vi "Initalize SR830(SubVI).vi"(0 "簇":T1={"initialize"=enum."SR830", "6221"={"6221 Resource"="GPIB0::24::INSTR", "Delta status"=FALSE, "电流"=0.0}, "SR830+6221"={"source"=0, "阻抗"=0.0, "量程入 4"=0, "量程入 3"=0, "量程入 2"=0, "量程入 1"=0, "SR830 2"=FALSE, "SR830 3"=FALSE, "SR830 4"=FALSE, "SR830 1"=FALSE, "VISA 1"="", "VISA 2"="", "VISA 3"="", "VISA 4"="", "量程"=enum."量程每次测量会判定"}, "2400"={"2400"=FALSE, "VISA"=""}, "ch"={"ch"=[], "current"=[], "change?"=[], "holding current\nwhen change ch?"=FALSE}, "Instrument"={"335 Resource"="GPIB0::24::INSTR", "Input (0:A)"=0, "Instrument Type"=enum."SVSM", "quantum design"=refnum, "Heater Output (1:1)"=1, "semaphore"=refnum, "TCP master instance"=refnum, "335 Status"=refnum, "M24C Resource"="GPIB0::24::INSTR", "4G supply"="GPIB0::24::INSTR", "Temp Status 24C"=refnum, "4g supply status"=refnum}, "Aborting"=refnum, "数据文件"=refnum} {"Instrument"."Input (0:A)" items=["A", "B"]; "Instrument"."Heater Output (1:1)" items=["1"=1, "2"=2]; "SR830+6221"."source" items=["SR830 1", "SR830 2", "SR830 3", "SR830 4"]}, 9 "字符串":string) -> (4 "输出簇":T1={"initialize"=enum."SR830", "6221"={"6221 Resource"="GPIB0::24::INSTR", "Delta status"=FALSE, "电流"=0.0}, "SR830+6221"={"source"=0, "阻抗"=0.0, "量程入 4"=0, "量程入 3"=0, "量程入 2"=0, "量程入 1"=0, "SR830 2"=FALSE, "SR830 3"=FALSE, "SR830 4"=FALSE, "SR830 1"=FALSE, "VISA 1"="", "VISA 2"="", "VISA 3"="", "VISA 4"="", "量程"=enum."量程每次测量会判定"}, "2400"={"2400"=FALSE, "VISA"=""}, "ch"={"ch"=[], "current"=[], "change?"=[], "holding current\nwhen change ch?"=FALSE}, "Instrument"={"335 Resource"="GPIB0::24::INSTR", "Input (0:A)"=0, "Instrument Type"=enum."SVSM", "quantum design"=refnum, "Heater Output (1:1)"=1, "semaphore"=refnum, "TCP master instance"=refnum, "335 Status"=refnum, "M24C Resource"="GPIB0::24::INSTR", "4G supply"="GPIB0::24::INSTR", "Temp Status 24C"=refnum, "4g supply status"=refnum}, "Aborting"=refnum, "数据文件"=refnum} {"Instrument"."Input (0:A)" items=["A", "B"]; "Instrument"."Heater Output (1:1)" items=["1"=1, "2"=2]; "SR830+6221"."source" items=["SR830 1", "SR830 2", "SR830 3", "SR830 4"]})   [LabVIEW 2019, in "SubVI.lvlib"]
uses:
  SubVI.lvlib
  lib/Keithley 622x/Configure/6221 Wave/Typedefs/KE6221 -- Wave Sine Wave Params.ctl
  lib/Keithley 622x/Configure/6221 Wave/Low Level/Typedefs/KE6221 -- Wave Frequency.ctl
  lib/Keithley 622x/Configure/6221 Wave/Low Level/Typedefs/KE6221 -- Wave Amplitude.ctl
  lib/Keithley 622x/Configure/Source/Typedefs/KE622x -- Current Level.ctl
  lib/Keithley 622x/Configure/6221 Wave/Low Level/Typedefs/KE6221 -- Wave Ranging Mode.ctl
  lib/Keithley 622x/Configure/Source/Typedefs/KE622x -- Current Ranges.ctl
  lib/Keithley 622x/Configure/6221 Wave/Low Level/Typedefs/KE6221 -- Wave Playback Mode.ctl
  lib/Keithley 622x/Configure/6221 Wave/Low Level/Typedefs/KE6221 -- Wave Playback Time.ctl
  lib/Keithley 622x/Configure/6221 Wave/Low Level/Typedefs/KE6221 -- Wave Playback Num Cycles.ctl
  lib/Keithley 622x/Configure/6221 Wave/Low Level/Typedefs/KE6221 -- Wave Phase Marker.ctl
  lib/Keithley 622x/Configure/Trigger/Low Level/Typedefs/KE622x -- Trig Link Line.ctl
  config.ctl
  <vilib>/NI/Modbus Library/API/Master/Modbus Master.lvclass
  initialize.ctl
  Instrument.ctl
  Instrument Type.ctl
  lib/QDInstrument.dll
  335 state.ctl
  lib/Keithley 622x/Configure/6221 Wave/Low Level/Typedefs/KE6221 -- Wave Type.ctl
  lib/Keithley 622x/Keithley 622x.lvlib
panel:
  in  "同步 3":bool
  in  "同步 2":bool
  in  "同步":bool
  in  "6221(SR830做源可忽略）":T17={"Sine Wave Params In"={"Frequency (Hz)"=1000.0, "Amplitude (A)"=0.001, "Offset (A)"=0.0, "Ranging Mode"=enum."Best", "Fixed Range"=enum."2mA", "Playback Mode"=enum."Time", "Time (s)"=999999.999, "Num Cycles"=1.0, "Phase\nMarker?"=FALSE, "Phase Marker (deg)"=180.0, "Trig Link Line"=enum."1"}, "RMS Amplitude (A)"=0.001, "6221 resource"=""} {"RMS Amplitude (A)" min=2e-12 max=0.105 format="%.3p"; "Sine Wave Params In"."Offset (A)" min=-0.105 max=0.105 format="%.4p"; "Sine Wave Params In"."Num Cycles" min=0.001 max=99999999900.0 format="%.3p"; "Sine Wave Params In"."Time (s)" min=1e-07 max=999999.999 format="%.3p"; "Sine Wave Params In"."Phase Marker (deg)" min=0.0 max=360.0 format="%.3f"; "Sine Wave Params In"."Amplitude (A)" min=2e-12 max=0.105 format="%.3p"; "Sine Wave Params In"."Frequency (Hz)" min=0.001 max=100000.0 format="%.3p"}
  in  "仪器设置":T18={"ID Query"=FALSE, "Reset"=FALSE, "VISA 1"="", "VISA 2"="", "VISA 3"="", "VISA 4"="", "Sensitivity 2"=-1, "Sensitivity 1"=-1, "量程"=enum."量程每次测量会判定", "SR830源配合的阻抗（6221做源可忽略）"=0.0, "SR830 2"=FALSE, "SR830 3"=FALSE, "SR830 4"=FALSE, "Sensitivity 3"=-1, "Sensitivity 4"=-1, "source"=0, "SR830 1"=FALSE} {"source" items=["SR830 1", "SR830 2", "SR830 3", "SR830 4", "6221"]; "Sensitivity 4" items=["Auto Gain"=-1, "2 nV/fA"=0, "5 nV/fA"=1, "10 nV/fA"=2, "20 nV/fA"=3, "50 nV/fA"=4, "100 nV/fA"=5, "200 nV/fA"=6, "500 nV/fA"=7, "1 uV/pA"=8, "2 uV/pA"=9, "5 uV/pA"=10, "10 uV/pA"=11, "20 uV/pA"=12, "50 uV/pA"=13, "100 uV/pA"=14, "200 uV/pA"=15, "500 uV/pA"=16, "1 mV/nA"=17, "2 mV/nA"=18, "5 mV/nA"=19, "10 mV/nA"=20, "20 mV/nA"=21, "50 mV/nA"=22, "100 mV/nA"=23, "200 mV/nA"=24, "500 mV/mA"=25, "1 V/uA"=26]; "Sensitivity 3" items=["Auto Gain"=-1, "2 nV/fA"=0, "5 nV/fA"=1, "10 nV/fA"=2, "20 nV/fA"=3, "50 nV/fA"=4, "100 nV/fA"=5, "200 nV/fA"=6, "500 nV/fA"=7, "1 uV/pA"=8, "2 uV/pA"=9, "5 uV/pA"=10, "10 uV/pA"=11, "20 uV/pA"=12, "50 uV/pA"=13, "100 uV/pA"=14, "200 uV/pA"=15, "500 uV/pA"=16, "1 mV/nA"=17, "2 mV/nA"=18, "5 mV/nA"=19, "10 mV/nA"=20, "20 mV/nA"=21, "50 mV/nA"=22, "100 mV/nA"=23, "200 mV/nA"=24, "500 mV/mA"=25, "1 V/uA"=26]; "Sensitivity 1" items=["Auto Gain"=-1, "2 nV/fA"=0, "5 nV/fA"=1, "10 nV/fA"=2, "20 nV/fA"=3, "50 nV/fA"=4, "100 nV/fA"=5, "200 nV/fA"=6, "500 nV/fA"=7, "1 uV/pA"=8, "2 uV/pA"=9, "5 uV/pA"=10, "10 uV/pA"=11, "20 uV/pA"=12, "50 uV/pA"=13, "100 uV/pA"=14, "200 uV/pA"=15, "500 uV/pA"=16, "1 mV/nA"=17, "2 mV/nA"=18, "5 mV/nA"=19, "10 mV/nA"=20, "20 mV/nA"=21, "50 mV/nA"=22, "100 mV/nA"=23, "200 mV/nA"=24, "500 mV/mA"=25, "1 V/uA"=26]; "Sensitivity 2" items=["Auto Gain"=-1, "2 nV/fA"=0, "5 nV/fA"=1, "10 nV/fA"=2, "20 nV/fA"=3, "50 nV/fA"=4, "100 nV/fA"=5, "200 nV/fA"=6, "500 nV/fA"=7, "1 uV/pA"=8, "2 uV/pA"=9, "5 uV/pA"=10, "10 uV/pA"=11, "20 uV/pA"=12, "50 uV/pA"=13, "100 uV/pA"=14, "200 uV/pA"=15, "500 uV/pA"=16, "1 mV/nA"=17, "2 mV/nA"=18, "5 mV/nA"=19, "10 mV/nA"=20, "20 mV/nA"=21, "50 mV/nA"=22, "100 mV/nA"=23, "200 mV/nA"=24, "500 mV/mA"=25, "1 V/uA"=26]}
  out "错误输出":errorcluster
  in  "滤波设置 4":T19={"Time Constant "=8, "Low Pass Filter Slope "=1, "Enable Sync Filter "=TRUE} {"Low Pass Filter Slope" items=["6 dB/oct", "12 dB/oct", "18 db/oct", "24 dB/oct"]; "Time Constant" items=["10 us", "30 us", "100 us", "300 us", "1 ms", "3 ms", "10 ms", "30 ms", "100 ms", "300 ms", "1 s", "3 s", "10 s", "30 s", "100 s", "300 s", "1 ks", "3 ks", "10 ks", "30 ks"]}
  in  "滤波设置 3":T19={"Time Constant "=8, "Low Pass Filter Slope "=1, "Enable Sync Filter "=TRUE} {"Low Pass Filter Slope" items=["6 dB/oct", "12 dB/oct", "18 db/oct", "24 dB/oct"]; "Time Constant" items=["10 us", "30 us", "100 us", "300 us", "1 ms", "3 ms", "10 ms", "30 ms", "100 ms", "300 ms", "1 s", "3 s", "10 s", "30 s", "100 s", "300 s", "1 ks", "3 ks", "10 ks", "30 ks"]}
  in  "滤波设置 2":T19={"Time Constant "=8, "Low Pass Filter Slope "=1, "Enable Sync Filter "=TRUE} {"Low Pass Filter Slope" items=["6 dB/oct", "12 dB/oct", "18 db/oct", "24 dB/oct"]; "Time Constant" items=["10 us", "30 us", "100 us", "300 us", "1 ms", "3 ms", "10 ms", "30 ms", "100 ms", "300 ms", "1 s", "3 s", "10 s", "30 s", "100 s", "300 s", "1 ks", "3 ks", "10 ks", "30 ks"]}
  in  "参考信号 4":T20={"Reference Source"=1, "External Reference Trigger  "=0, "Detection Harmonic Number "=1.0, "Manual Phase (Degree)"=0.0, "Auto Phase "=FALSE, "Sine Output Amplitude (V)"=1.0, "Internal Reference Frequency (Hz)"=13.0} {"External Reference Trigger" items=["Sine Zero Crossing", "TTL Rising Edge", "TTL Falling Edge"]; "Reference Source" items=["External", "Internal"]}
  in  "参考信号 3":T20={"Reference Source"=1, "External Reference Trigger  "=0, "Detection Harmonic Number "=1.0, "Manual Phase (Degree)"=0.0, "Auto Phase "=FALSE, "Sine Output Amplitude (V)"=1.0, "Internal Reference Frequency (Hz)"=13.0} {"External Reference Trigger" items=["Sine Zero Crossing", "TTL Rising Edge", "TTL Falling Edge"]; "Reference Source" items=["External", "Internal"]}
  in  "参考信号 2":T20={"Reference Source"=1, "External Reference Trigger  "=0, "Detection Harmonic Number "=1.0, "Manual Phase (Degree)"=0.0, "Auto Phase "=FALSE, "Sine Output Amplitude (V)"=1.0, "Internal Reference Frequency (Hz)"=13.0} {"External Reference Trigger" items=["Sine Zero Crossing", "TTL Rising Edge", "TTL Falling Edge"]; "Reference Source" items=["External", "Internal"]}
  in  "输入信号 4":T21={"Input Notch Filter "=0, "Input Shield Grounding"=0, "Input Coupling "=0, "Input Connection  "=1} {"Input Connection" items=["Single-Ended Voltage", "Differential Voltage", "1 MOhm Current Gain", "100 MOhm Current Gain"]; "Input Coupling" items=["AC", "DC"]; "Input Shield Grounding" items=["Float", "Ground"]; "Input Notch Filter" items=["None", "Line Notch", "2x Line Notch", "Both Notch Filters"]}
  in  "输入信号 3":T21={"Input Notch Filter "=0, "Input Shield Grounding"=0, "Input Coupling "=0, "Input Connection  "=1} {"Input Connection" items=["Single-Ended Voltage", "Differential Voltage", "1 MOhm Current Gain", "100 MOhm Current Gain"]; "Input Coupling" items=["AC", "DC"]; "Input Shield Grounding" items=["Float", "Ground"]; "Input Notch Filter" items=["None", "Line Notch", "2x Line Notch", "Both Notch Filters"]}
  in  "输入信号 2":T21={"Input Notch Filter "=0, "Input Shield Grounding"=0, "Input Coupling "=0, "Input Connection  "=1} {"Input Connection" items=["Single-Ended Voltage", "Differential Voltage", "1 MOhm Current Gain", "100 MOhm Current Gain"]; "Input Coupling" items=["AC", "DC"]; "Input Shield Grounding" items=["Float", "Ground"]; "Input Notch Filter" items=["None", "Line Notch", "2x Line Notch", "Both Notch Filters"]}
  in  "滤波设置":T19={"Time Constant "=8, "Low Pass Filter Slope "=1, "Enable Sync Filter "=TRUE} {"Low Pass Filter Slope" items=["6 dB/oct", "12 dB/oct", "18 db/oct", "24 dB/oct"]; "Time Constant" items=["10 us", "30 us", "100 us", "300 us", "1 ms", "3 ms", "10 ms", "30 ms", "100 ms", "300 ms", "1 s", "3 s", "10 s", "30 s", "100 s", "300 s", "1 ks", "3 ks", "10 ks", "30 ks"]}
  in  "参考信号":T20={"Reference Source"=1, "External Reference Trigger  "=0, "Detection Harmonic Number "=1.0, "Manual Phase (Degree)"=0.0, "Auto Phase "=FALSE, "Sine Output Amplitude (V)"=1.0, "Internal Reference Frequency (Hz)"=13.0} {"External Reference Trigger" items=["Sine Zero Crossing", "TTL Rising Edge", "TTL Falling Edge"]; "Reference Source" items=["External", "Internal"]}
  in  "输入信号":T21={"Input Notch Filter "=0, "Input Shield Grounding"=0, "Input Coupling "=0, "Input Connection  "=1} {"Input Connection" items=["Single-Ended Voltage", "Differential Voltage", "1 MOhm Current Gain", "100 MOhm Current Gain"]; "Input Coupling" items=["AC", "DC"]; "Input Shield Grounding" items=["Float", "Ground"]; "Input Notch Filter" items=["None", "Line Notch", "2x Line Notch", "Both Notch Filters"]}
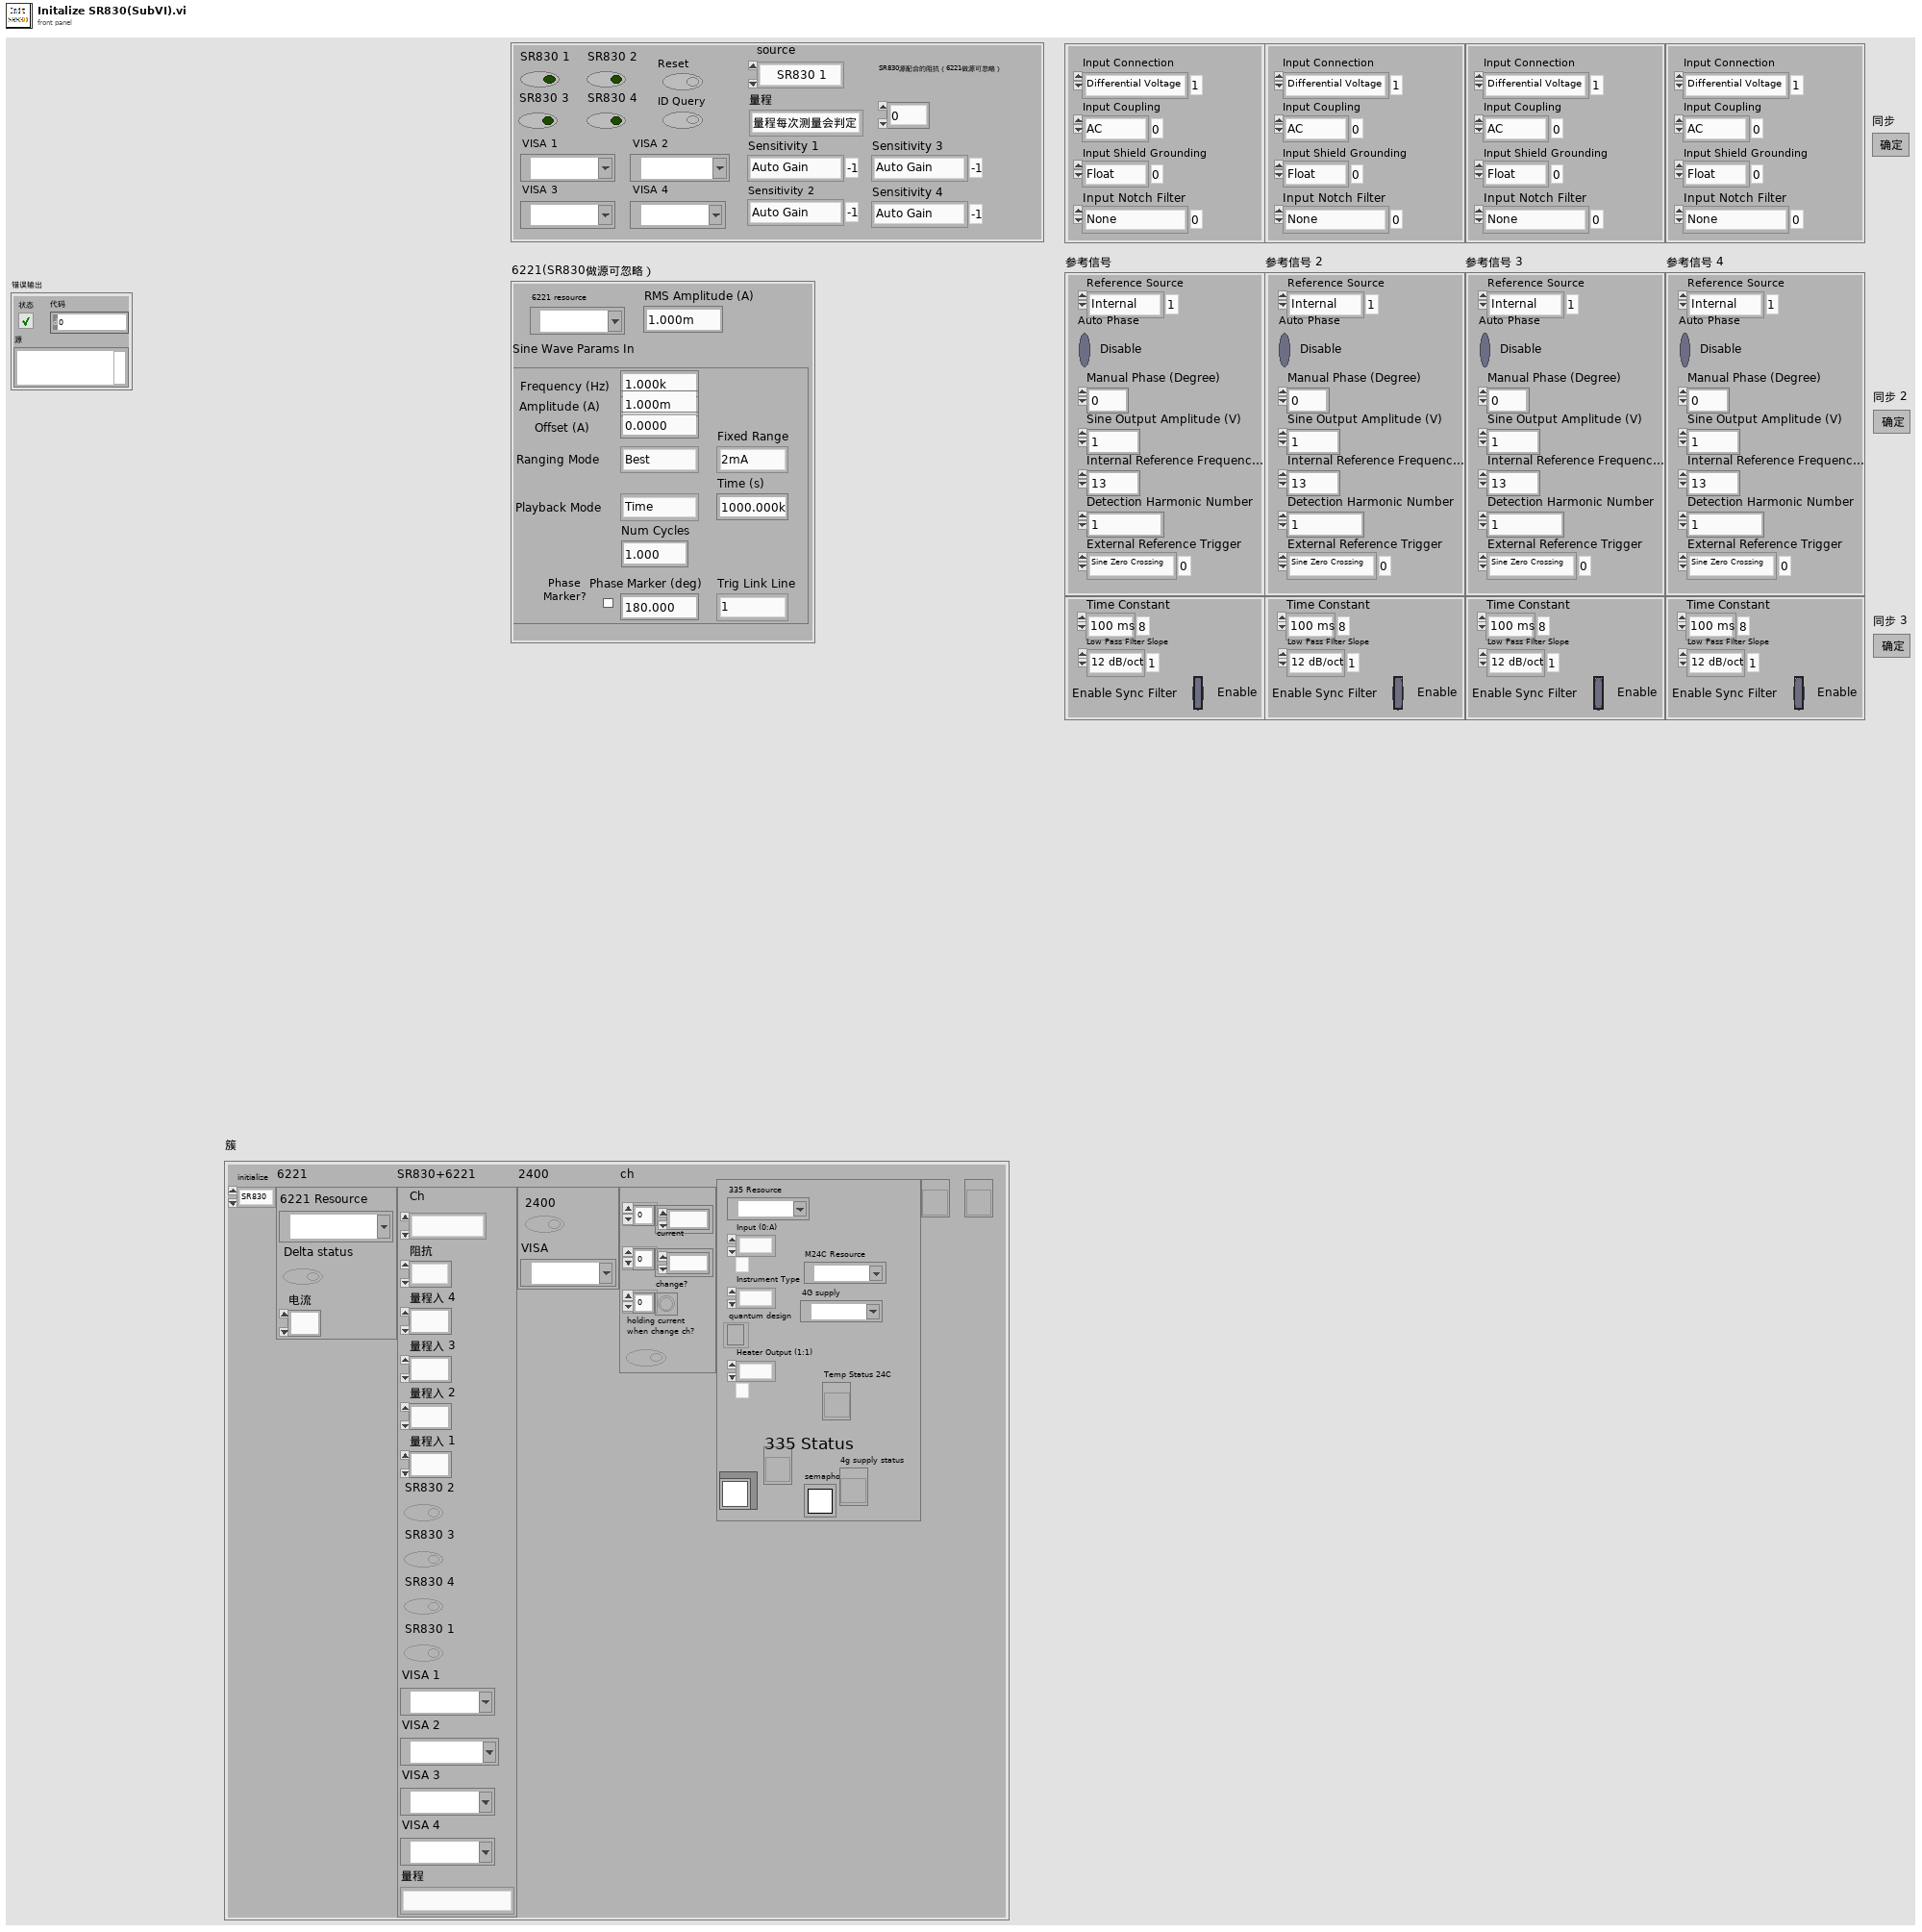
[diagram p1: front panel]
types:
  T1 = typedef "config.ctl" = cluster{"initialize":T2, "6221":cluster{"6221 Resource":refnum<visa-resource-name>, "Delta status":bool, "电流":dbl}, "SR830+6221":cluster{"source":u16, "阻抗":dbl, "量程入 4":i32, "量程入 3":i32, "量程入 2":i32, "量程入 1":i32, "SR830 2":bool, "SR830 3":bool, "SR830 4":bool, "SR830 1":bool, "VISA 1":refnum<visa-resource-name>, "VISA 2":refnum<visa-resource-name>, "VISA 3":refnum<visa-resource-name>, "VISA 4":refnum<visa-resource-name>, "量程":enum16{"量程每次测量会判定", "量程不变为设定值"}}, "2400":cluster{"2400":bool, "VISA":refnum<visa-resource-name>}, "ch":cluster{"ch":i32[], "current":dbl[], "change?":bool[], "holding current\nwhen change ch?":bool}, "Instrument":T3, "Aborting":refnum<vi>, "数据文件":refnum<vi>}
  T2 = typedef "initialize.ctl" = enum16{"SR830", "keithley6221-SR830", "Delta", "Delta-tunnelling", "keithley6221-2182-DC"}
  T3 = typedef "Instrument.ctl" = cluster{"335 Resource":refnum<visa-resource-name>, "Input (0:A)":u16, "Instrument Type":T4, "quantum design":refnum<k24>, "Heater Output (1:1)":u16, "semaphore":T5, "TCP master instance":refnum<class "Modbus Master.lvclass">, "335 Status":refnum<vi>, "M24C Resource":refnum<visa-resource-name>, "4G supply":refnum<visa-resource-name>, "Temp Status 24C":refnum<vi>, "4g supply status":refnum<vi>}
  T4 = typedef "Instrument Type.ctl" = enum16{"PPMS", "VersaLab", "DynaCool", "SVSM", "PPMS-Rotate", "Lakeshore335", "9T mag"}
  T5 = typedef "Semaphore RefNum" = refnum<k1>
  T6 = typedef "Keithley 622x.lvlib/KE6221 -- Wave Sine Wave Params.ctl" = cluster{"Frequency (Hz)":T7, "Amplitude (A)":T8, "Offset (A)":T9, "Ranging Mode":T10, "Fixed Range":T11, "Playback Mode":T12, "Time (s)":T13, "Num Cycles":T14, "Phase\nMarker?":bool, "Phase Marker (deg)":T15, "Trig Link Line":T16}
  T7 = typedef "Keithley 622x.lvlib/KE6221 -- Wave Frequency.ctl" = dbl
  T8 = typedef "Keithley 622x.lvlib/KE6221 -- Wave Amplitude.ctl" = dbl
  T9 = typedef "Keithley 622x.lvlib/KE622x -- Current Level.ctl" = dbl
  T10 = typedef "Keithley 622x.lvlib/KE6221 -- Wave Ranging Mode.ctl" = enum16{"Best", "Fixed"}
  T11 = typedef "Keithley 622x.lvlib/KE622x -- Current Ranges.ctl" = enum16{"2nA", "20nA", "200nA", "2uA", "20uA", "200uA", "2mA", "20mA", "100mA"}
  T12 = typedef "Keithley 622x.lvlib/KE6221 -- Wave Playback Mode.ctl" = enum16{"Time", "Num Cycles"}
  T13 = typedef "Keithley 622x.lvlib/KE6221 -- Wave Playback Time.ctl" = dbl
  T14 = typedef "Keithley 622x.lvlib/KE6221 -- Wave Playback Num Cycles.ctl" = dbl
  T15 = typedef "Keithley 622x.lvlib/KE6221 -- Wave Phase Marker.ctl" = dbl
  T16 = typedef "Keithley 622x.lvlib/KE622x -- Trig Link Line.ctl" = enum16{"1", "2", "3", "4", "5", "6"}
  T17 = cluster{"Sine Wave Params In":T6, "RMS Amplitude (A)":T8, "6221 resource":refnum<visa-resource-name>}
  T18 = cluster{"ID Query":bool, "Reset":bool, "VISA 1":refnum<visa-resource-name>, "VISA 2":refnum<visa-resource-name>, "VISA 3":refnum<visa-resource-name>, "VISA 4":refnum<visa-resource-name>, "Sensitivity 2":i16, "Sensitivity 1":i16, "量程":enum16{"量程每次测量会判定", "量程不变为设定值"}, "SR830源配合的阻抗（6221做源可忽略）":dbl, "SR830 2":bool, "SR830 3":bool, "SR830 4":bool, "Sensitivity 3":i16, "Sensitivity 4":i16, "source":u16, "SR830 1":bool}
  T19 = cluster{"Time Constant ":u16, "Low Pass Filter Slope ":u16, "Enable Sync Filter ":bool}
  T20 = cluster{"Reference Source":u16, "External Reference Trigger  ":u16, "Detection Harmonic Number ":dbl, "Manual Phase (Degree)":dbl, "Auto Phase ":bool, "Sine Output Amplitude (V)":dbl, "Internal Reference Frequency (Hz)":dbl}
  T21 = cluster{"Input Notch Filter ":u16, "Input Shield Grounding":u16, "Input Coupling ":u16, "Input Connection  ":u16}
  T22 = typedef "Keithley 622x.lvlib/KE6221 -- Wave Type.ctl" = enum16{"Sinusoid", "Square", "Ramp", "Arbitrary 0", "Arbitrary 1", "Arbitrary 2", "Arbitrary 3", "Arbitrary 4"}
  T23 = enum16{"open", "replace", "create", "open or create", "replace or create", "replace or create with confirmation"}
  T24 = typedef "Keithley 622x.lvlib/KE622x -- On Off Control.ctl" = enum16{"Off", "On"}
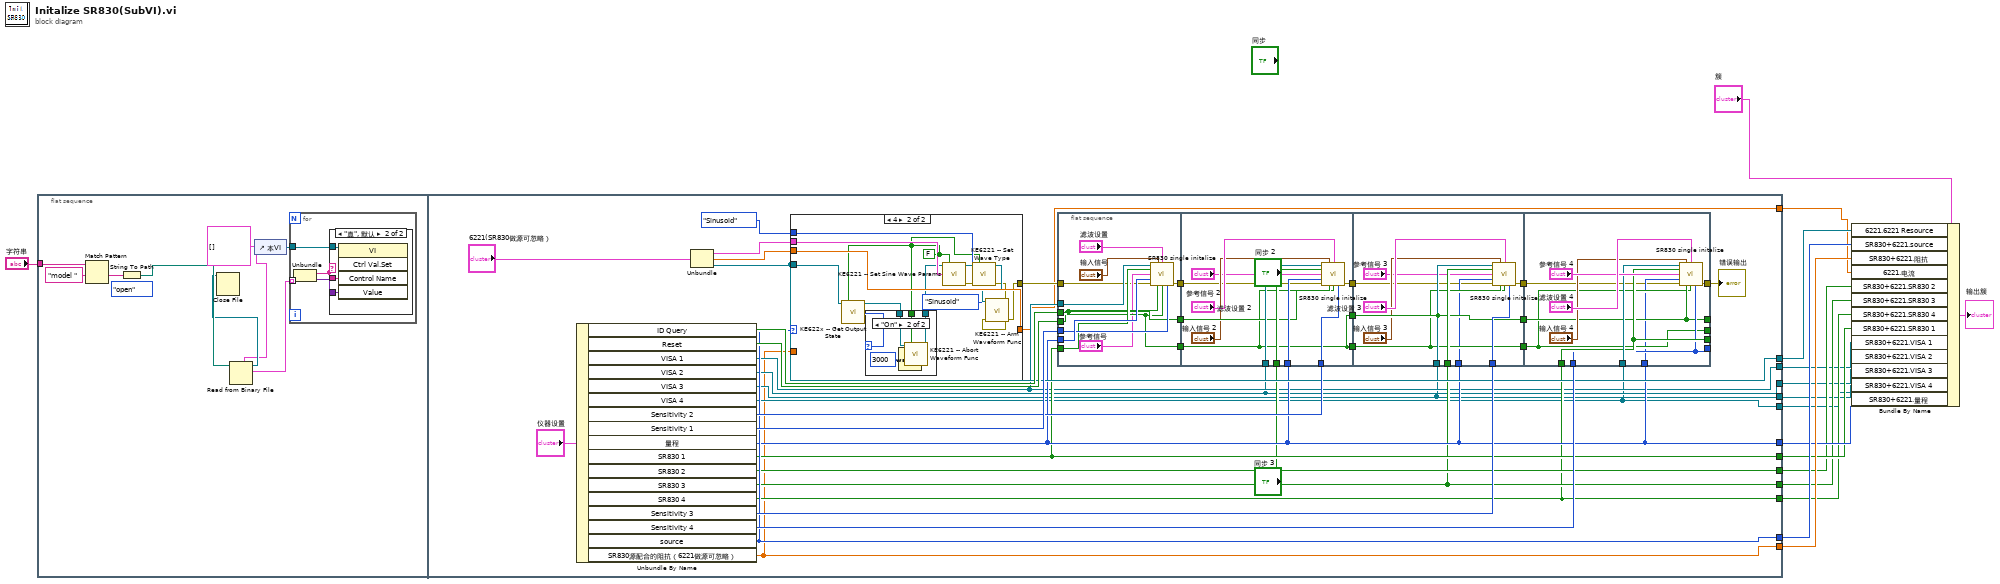
[diagram p0: block diagram]
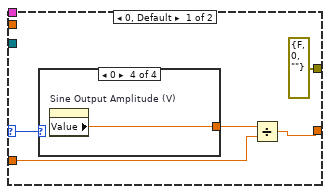
[diagram p3: hidden frame]
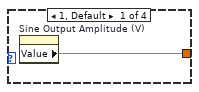
[diagram p4: hidden frame]
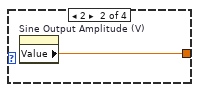
[diagram p5: hidden frame]
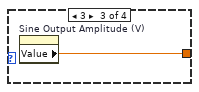
[diagram p6: hidden frame]
diagram:
  n1 = flat-sequence {
    tunnel: "字符串" -> [w24]
    tunnel: [w48] -> w14
    tunnel: [w45] -> w15
    tunnel: [w33] -> w13
    tunnel: [w43] -> w12
    tunnel: [w42] -> w11
    tunnel: [w41] -> w10
    tunnel: [w40] -> w9
    tunnel: [w39] -> w8
    tunnel: [w38] -> w7
    tunnel: [w37] -> w6
    tunnel: [w36] -> w5
    tunnel: [w35] -> w4
    tunnel: [w32] -> w3
    frame #0 {
      (unwired) T23."open" ("操作(0:open)")
      n2 = Match Pattern(string=w24, regular expression="model " ("正则表达式")) -> (after substring=w23:string)  [unwired: 1 in, 3 out]
      n3 = String To Path(string=w23) -> (path=w20:path)
      n4 = Read from Binary File(5:cluster{"Name":string, "Variant Data":variant}[] [] ("控件值:获取全部"), 11:w20) -> (2:w17:cluster{"Name":string, "Variant Data":variant}[], 3:w19:refnum<file>)  [unwired: 4 in, 2 out]
      n5 = Close File(refnum=w19) -> ()  [unwired: 1 in, 2 out]
      n6 = control-ref of="本VI"() -> (w21:refnum<vi>)
      n7 = for {
        tunnel: w17 -> [w28] mode=indexing
        tunnel: w21 -> [w27]
        n8 = Unbundle(w28) -> ("Name"=w25:string, "Variant Data"=w26:variant)
        n9 = case shown="\"真\", 默认" w25 {
          tunnel: w27 -> [_ w31]
          tunnel: w25 -> [_ w30]
          tunnel: w26 -> [_ w29]
          frame "6221", "cancel", "load", "model", "ok" {
          }
          frame "真", Default {
            n10 = invoke class="VI" method="Ctrl Val.Set"(reference=w31, "Control Name"=w30, "Value"=w29) -> ()  [unwired: 2 in, 5 out]
          }
        }
      }
    }
    frame #1 {
      n11 = Unbundle By Name("仪器设置") -> ("ID Query"=w65:bool, "Reset"=w64:bool, "VISA 1"=w38:refnum<visa-resource-name>, "VISA 2"=w37:refnum<visa-resource-name>, "VISA 3"=w36:refnum<visa-resource-name>, "VISA 4"=w35:refnum<visa-resource-name>, "Sensitivity 2"=w61:i16, "Sensitivity 1"=w66:i16, "量程"=w43:enum16{"量程每次测量会判定", "量程不变为设定值"}, "SR830 1"=w42:bool, "SR830 2"=w41:bool, "SR830 3"=w40:bool, "SR830 4"=w39:bool, "Sensitivity 3"=w63:i16, "Sensitivity 4"=w62:i16, "source"=w48:u16, "SR830源配合的阻抗（6221做源可忽略）"=w33:dbl)
      n12 = Unbundle("6221(SR830做源可忽略）") -> ("Sine Wave Params In"=w46:T6, "RMS Amplitude (A)"=w34:T8, "6221 resource"=w45:refnum<visa-resource-name>)
      n13 = case shown="4" w48 {
        selector: w48 -> [w68 _]
        tunnel: KE6221_--_Wave_Type."Sinusoid" ("Wave Type") -> [_ w89]
        tunnel: [errorcluster {"status"=FALSE, "code"=0, "source"=""} ("error out") w82] -> w49
        tunnel: w46 -> [_ w86]
        tunnel: w45 -> [_ w81]
        tunnel: w34 -> [_ w85]
        tunnel: w33 -> [w69 _]
        tunnel: [w67 w85] -> w32
        frame 0, Default {
          n14 = case shown="0" w68 {
            tunnel: [w72 w73 w74 w75] -> w70
            frame 1, Default {
              n15 = property on="Sine Output Amplitude (V)" class="DigNum (严格)"() -> ("Value"=w72:dbl)  [unwired: 2 in, 2 out]
            }
            frame 2 {
              n16 = property on="Sine Output Amplitude (V)" class="DigNum (严格)"() -> ("Value"=w73:dbl)  [unwired: 2 in, 2 out]
            }
            frame 3 {
              n17 = property on="Sine Output Amplitude (V)" class="DigNum (严格)"() -> ("Value"=w74:dbl)  [unwired: 2 in, 2 out]
            }
            frame 0 {
              n18 = property on="Sine Output Amplitude (V)" class="DigNum (严格)"() -> ("Value"=w75:dbl)  [unwired: 2 in, 2 out]
            }
          }
          n19 = Divide(x=w70, y=w69) -> (x/y=w67:dbl)
        }
        frame 4 {
          w78 = FALSE ("Check For SCPI Errors? (T)")
          n20 = call "KE622x -- Get Output State.vi"("Resource In"=w81, "Check For SCPI Errors? (T)"=w78) -> ("Resource Out (dupl)"=w79:refnum<visa-resource-name>, "Output State"=w80:T24)  [unwired: 11 in, 1 out]
          n21 = case shown="\"On\"" w80 {
            tunnel: w79 -> [w90 w94]
            tunnel: w78 -> [_ w93]
            tunnel: [w90 w92] -> w77
            frame "Off", Default {
            }
            frame "On" {
              n22 = Wait (ms)(milliseconds to wait=u32 3000 ("等待时间（毫秒）")) -> ()  [unwired: 1 out]
              n23 = call "KE6221 -- Abort Waveform Func.vi"("Resource In"=w94, "Check For SCPI Errors? (T)"=w93) -> ("Resource Out (dupl)"=w92:refnum<visa-resource-name>)  [unwired: 12 in, 1 out]
            }
          }
          n24 = call "KE6221 -- Set Sine Wave Params.vi"("Resource In"=w77, "Check For SCPI Errors? (T)"=w78, "Sine Wave Params In"=w86) -> ("Resource Out (dupl)"=w88:refnum<visa-resource-name>, "error out"=w87:errorcluster)  [unwired: 10 in, 1 out]
          n25 = call "KE6221 -- Set Wave Type.vi"("Resource In"=w88, "Check For SCPI Errors? (T)"=w78, "Wave Type"=w89, "error in (no error)"=w87) -> ("Resource Out (dupl)"=w84:refnum<visa-resource-name>, "error out"=w83:errorcluster)  [unwired: 10 in]
          n26 = call "KE6221 -- Arm Waveform Func.vi"("Resource In"=w84, "Wave Type"=KE6221_--_Wave_Type."Sinusoid", "error in (no error)"=w83) -> ("error out"=w82:errorcluster)  [unwired: 11 in, 1 out]
        }
      }
      n27 = flat-sequence {
        tunnel: w38 -> [w105]
        tunnel: w43 -> [w104]
        tunnel: w66 -> [w103]
        tunnel: w65 -> [w101]
        tunnel: w64 -> [w100]
        tunnel: w42 -> [w102]
        tunnel: [w101] -> w60
        tunnel: [w100] -> w59
        tunnel: [w96] -> w54
        tunnel: w49 -> [w95]
        tunnel: w37 -> [w116]
        tunnel: w41 -> [w115]
        tunnel: w61 -> [w114]
        tunnel: w43 -> [w113]
        tunnel: w60 -> [w112]
        tunnel: w59 -> [w111]
        tunnel: [w111] -> w58
        tunnel: [w111] -> w57
        tunnel: w54 -> [w107]
        tunnel: [w106] -> w53
        tunnel: w36 -> [w127]
        tunnel: w40 -> [w126]
        tunnel: w63 -> [w125]
        tunnel: w58 -> [w124]
        tunnel: w57 -> [w123]
        tunnel: [w124] -> w56
        tunnel: [w123] -> w55
        tunnel: w43 -> [w122]
        tunnel: w53 -> [w118]
        tunnel: [w117] -> w52
        tunnel: [w134] -> _
        tunnel: [w131] -> _
        tunnel: [w132] -> _
        tunnel: [w133] -> _
        tunnel: w35 -> [w135]
        tunnel: w39 -> [w134]
        tunnel: w62 -> [w133]
        tunnel: w56 -> [w132]
        tunnel: w55 -> [w131]
        tunnel: w43 -> [w130]
        tunnel: w52 -> [w129]
        tunnel: [w128] -> w51
        frame #0 {
          n28 = call "SR830 single initalize.vi"("VISA引用句柄输入"=w105, "输入信号"="输入信号", "滤波设置"="滤波设置", "open"=w102, "参考信号"="参考信号", "量程"=w104, "error in (no error)"=w95, "ID Query (True)"=w101, "Reset (True)"=w100, "Sensitivity (-1: Auto gain)"=w103) -> ("错误输出"=w96:cluster{"status":bool, "code":i32, string})  [unwired: 5 in]
        }
        frame #1 {
          n29 = call "SR830 single initalize.vi"("VISA引用句柄输入"=w116, "输入信号"="输入信号 2", "滤波设置"="滤波设置 2", "open"=w115, "参考信号"="参考信号 2", "量程"=w113, "error in (no error)"=w107, "ID Query (True)"=w112, "Reset (True)"=w111, "Sensitivity (-1: Auto gain)"=w114) -> ("错误输出"=w106:cluster{"status":bool, "code":i32, string})  [unwired: 5 in]
        }
        frame #2 {
          n30 = call "SR830 single initalize.vi"("VISA引用句柄输入"=w127, "输入信号"="输入信号 3", "滤波设置"="滤波设置 3", "open"=w126, "参考信号"="参考信号 3", "量程"=w122, "error in (no error)"=w118, "ID Query (True)"=w124, "Reset (True)"=w123, "Sensitivity (-1: Auto gain)"=w125) -> ("错误输出"=w117:cluster{"status":bool, "code":i32, string})  [unwired: 5 in]
        }
        frame #3 {
          n31 = call "SR830 single initalize.vi"("VISA引用句柄输入"=w135, "输入信号"="输入信号 4", "滤波设置"="滤波设置 4", "open"=w134, "参考信号"="参考信号 4", "量程"=w130, "error in (no error)"=w129, "ID Query (True)"=w132, "Reset (True)"=w131, "Sensitivity (-1: Auto gain)"=w133) -> ("错误输出"=w128:cluster{"status":bool, "code":i32, string})  [unwired: 5 in]
        }
      }
      "错误输出" <- w51
    }
  }
  n32 = Bundle By Name(cluster="簇", "6221.6221 Resource"=w15, "SR830+6221.source"=w14, "SR830+6221.阻抗"=w13, "6221.电流"=w3, "SR830+6221.SR830 2"=w10, "SR830+6221.SR830 3"=w9, "SR830+6221.SR830 4"=w8, "SR830+6221.SR830 1"=w11, "SR830+6221.VISA 1"=w7, "SR830+6221.VISA 2"=w6, "SR830+6221.VISA 3"=w5, "SR830+6221.VISA 4"=w4, "SR830+6221.量程"=w12) -> (→"输出簇":T1)
